vi "Sensor Scaling.vi"(8 "error in":errorcluster) -> (0 "error out":errorcluster, 3 "Output":cluster{"X":dbl[], "Y":dbl[], "Avg point":i16}[](array[cluster]))   [LabVIEW 2015]
uses:
  <vilib>/Analysis/NI_AALPro.lvlib
panel:
  in  "Avg Point":i16=1 min=1 max=500
  out "Offset":dbl format="%0.2f"
  out "Slope":dbl format="%0.2f"
  in  "Unit":string
  in  "Sensor":u16(ring) items=["Load Cell", "LVDT", "LOadcell1", "wq", "load3", "LVDT3", "gggh"]
  in  "Next":bool
  in  "Input Values":dbl[](array[numeric])
  in  "New Calibration":dbl[](array[numeric])
  in  "Sensor Add":bool
  in  "Graph Plot":bool
  in  "Help Button":bool
  in  "Quit":bool
  in  "Save":bool
  out "XY Graph":T1(graph)
  out "error out 2":errorcluster
  out "Numeric":dbl
  out "Old Calibration":dbl[](array[numeric])
  # "Sensor Calibration"
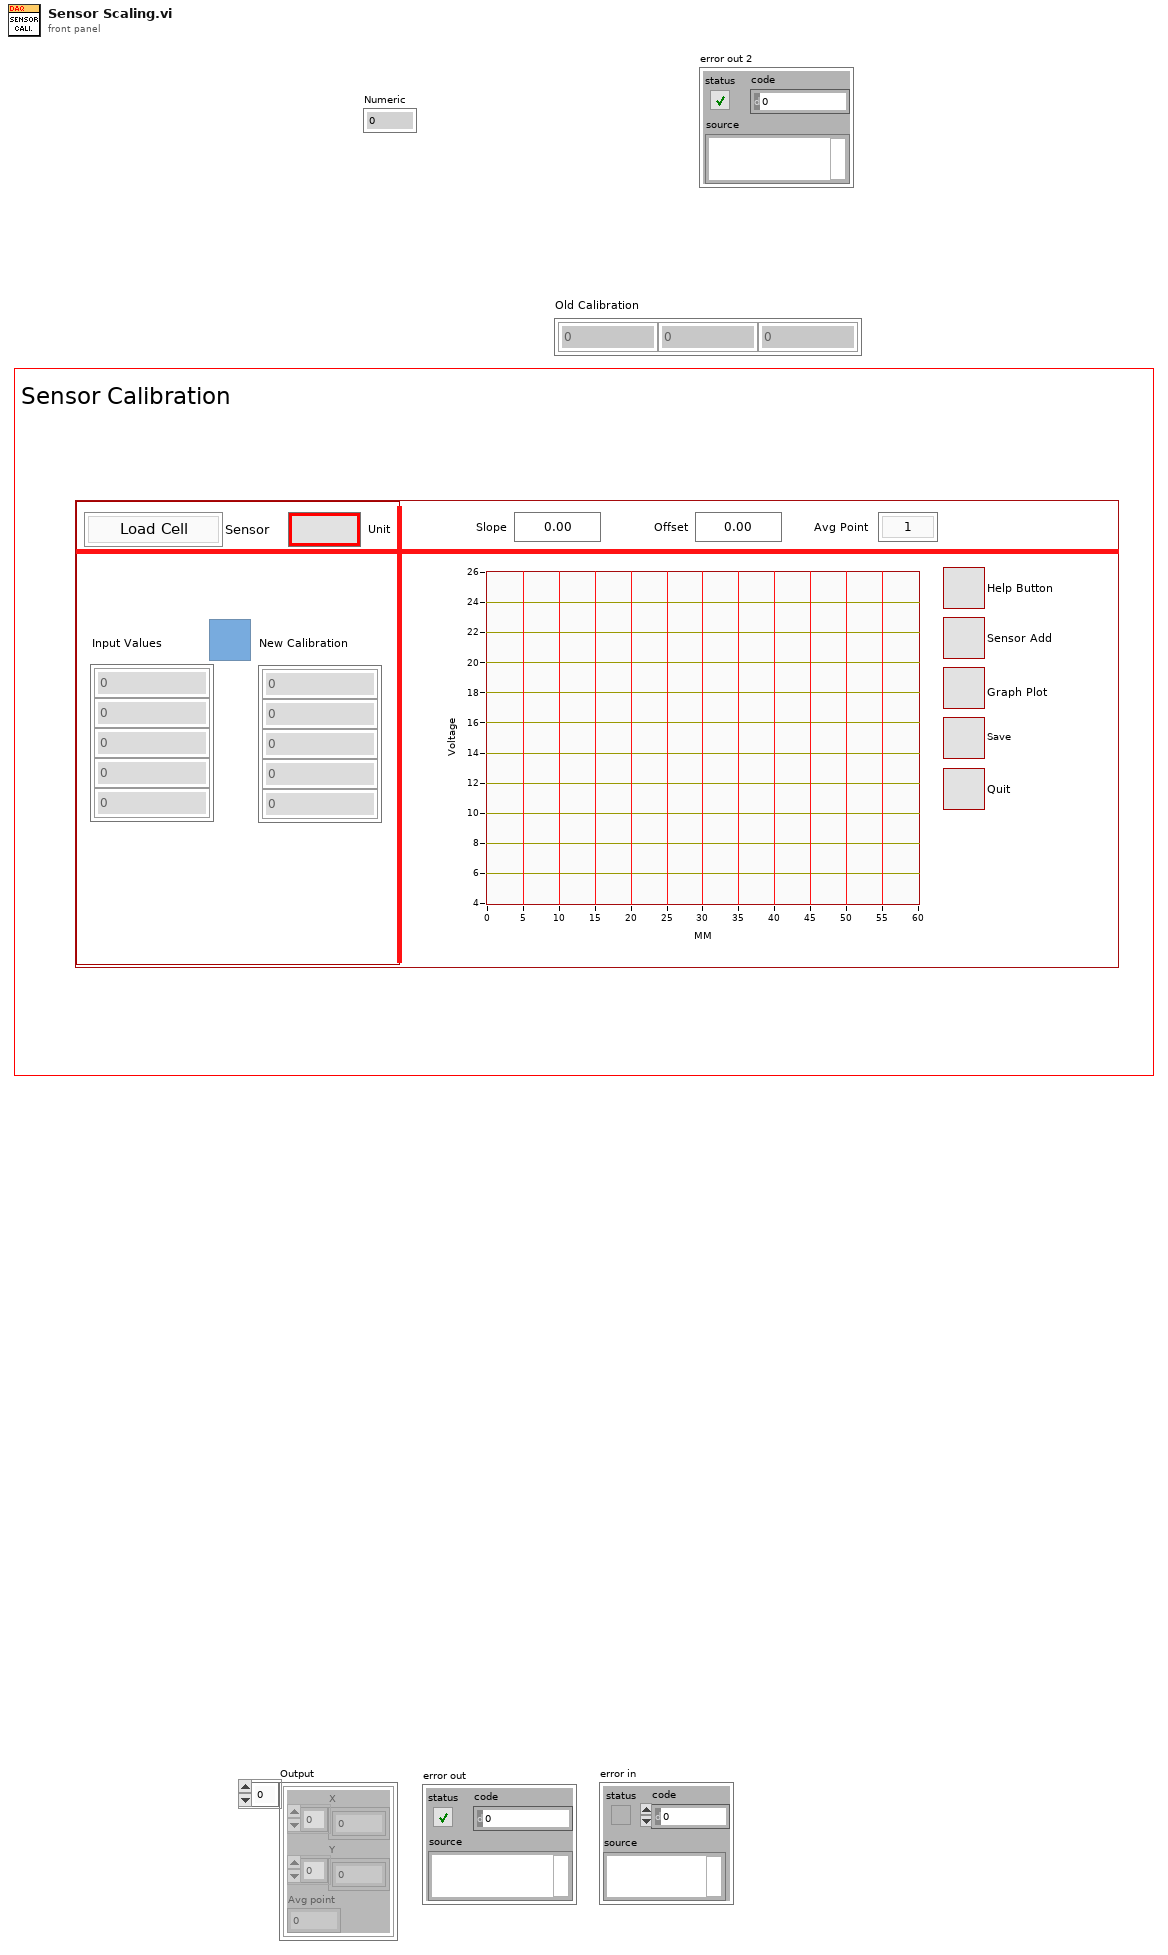
[diagram p1: front panel]
types:
  T1 = cluster{"Input Values":dbl[], "New Calibration":dbl[]}
  T2 = cluster{"XInput":dbl[], "Y New Value":dbl[], "Avg point":i16}[]
  T3 = cluster{"XInput":dbl[], "Y New Value":dbl[], "Avg point":i16}
  T4 = cluster{"Input Values":dbl[], "New Calibration":dbl[], "Sensor":u16}
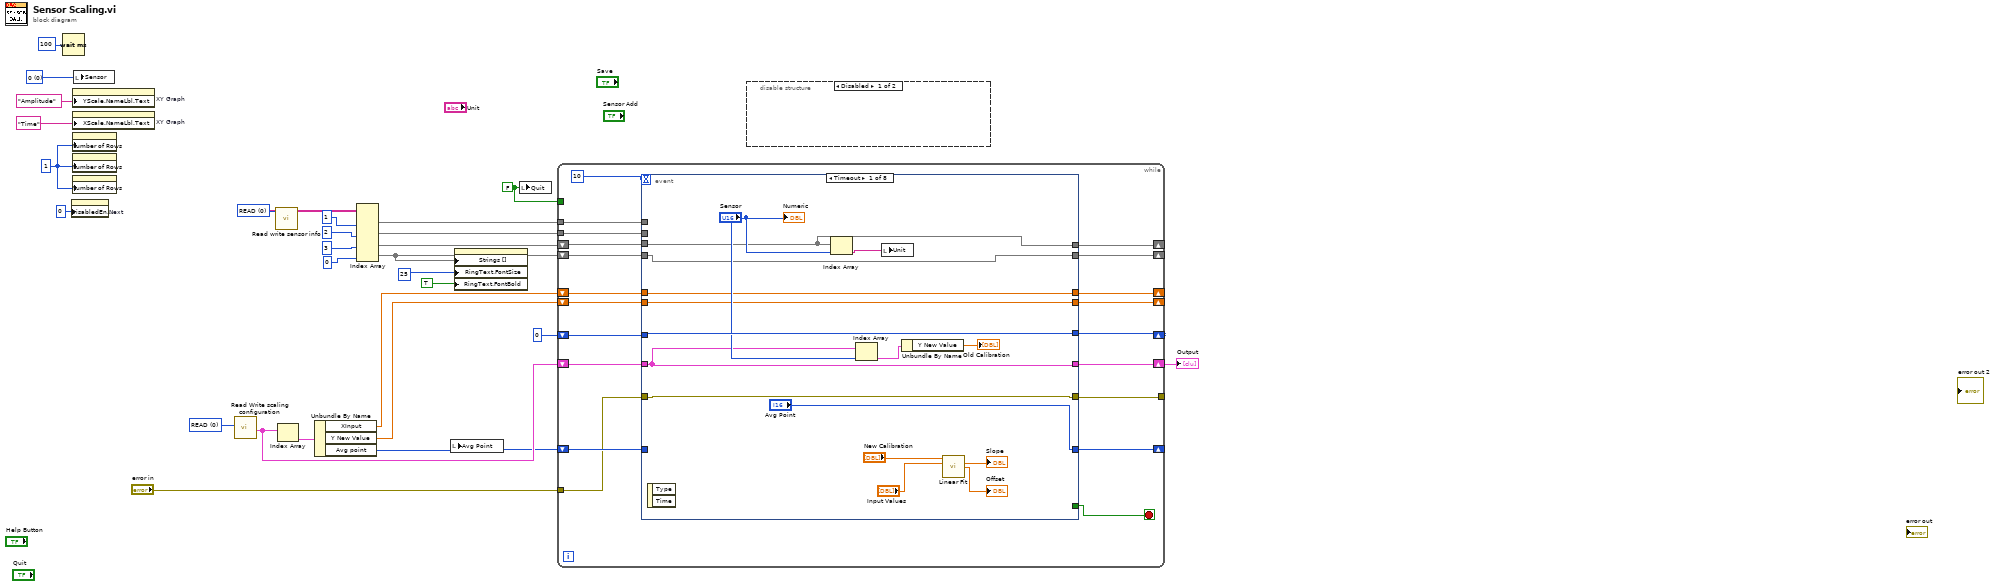
[diagram p0: block diagram]
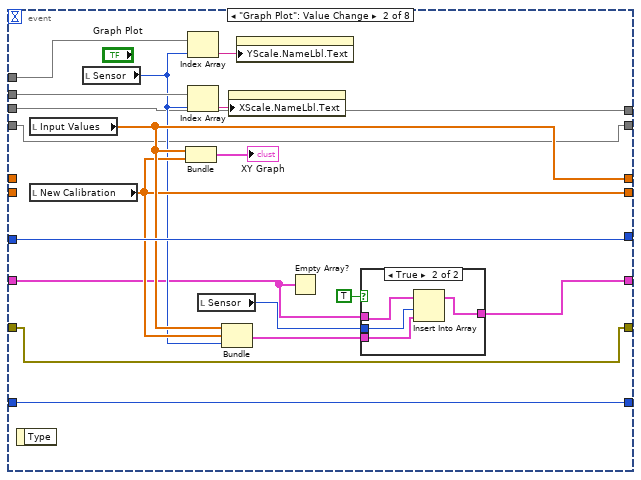
[diagram p3: hidden frame]
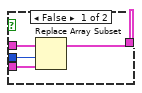
[diagram p4: hidden frame]
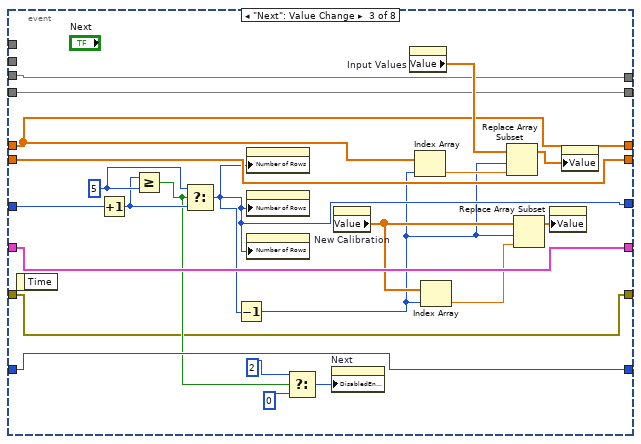
[diagram p5: hidden frame]
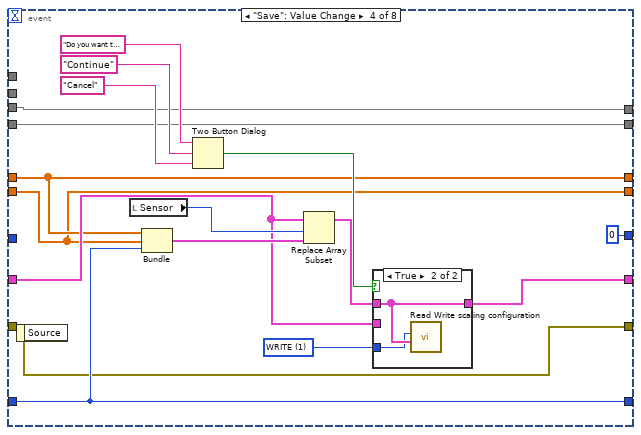
[diagram p6: hidden frame]
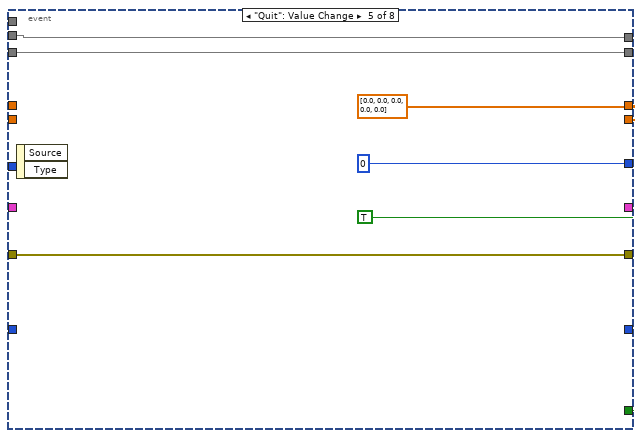
[diagram p8: hidden frame]
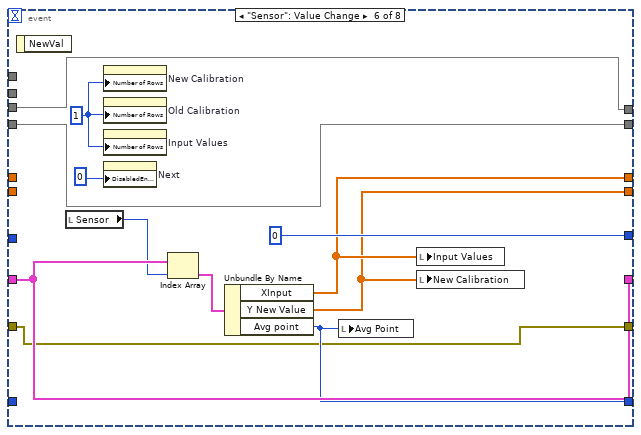
[diagram p9: hidden frame]
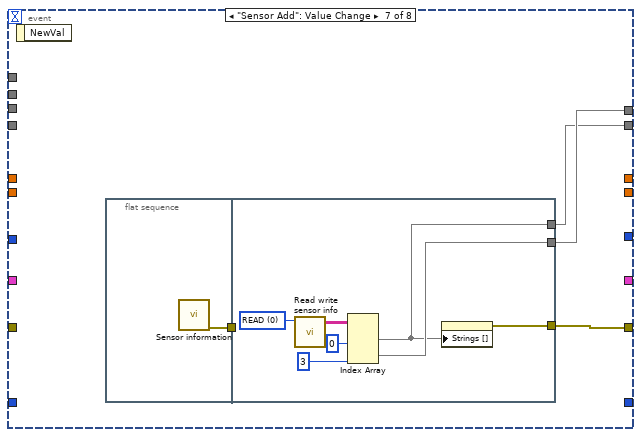
[diagram p10: hidden frame]
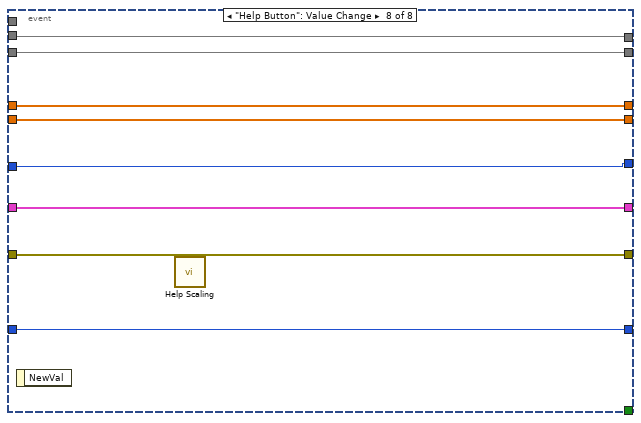
[diagram p11: hidden frame]
diagram:
  w3 = FALSE ("Quit")
  w13 = u16 0 items=["READ", "WRITE"] ("Read/Write")
  w19 = u16 0 items=["READ", "WRITE"] ("Read/Write")
  w9 = u32 1 ("Number of Rows")
  w27 = u16 0 items=["0", "1", "2", "3", "4", "5", "6", "7", "8", "9", "10", "11", "12", "13", "14", "15", "16", "17", "18", "19", "20", "21", "22", "23", "24", "25", "26", "27", "28", "29"] ("Ring")
  n1 = Wait (ms)(milliseconds to wait=u32 100) -> ()  [unwired: 1 out]
  n2 = property on="Next" class="Bool"("DisabledEnum"=u16 0) -> ()  [unwired: 2 in, 2 out]
  n3 = property on="XY Graph" class="XYGraph (strict)"("YScale.NameLbl.Text"="Amplitude" ("Y Scale.Name Label.Text")) -> ()  [unwired: 2 in, 2 out]
  n4 = property on="XY Graph" class="XYGraph (strict)"("XScale.NameLbl.Text"="Time" ("X Scale.Unit Label.Text")) -> ()  [unwired: 2 in, 2 out]
  n5 = property on="Old Calibration" class="Arr (strict)"("Number of Rows"=w9) -> ()  [unwired: 2 in, 2 out]
  n6 = property on="Input Values" class="Arr (strict)"("Number of Rows"=w9) -> ()  [unwired: 2 in, 2 out]
  n7 = property on="New Calibration" class="Arr (strict)"("Number of Rows"=w9) -> ()  [unwired: 2 in, 2 out]
  n8 = local write "Sensor"(w27) -> ()
  n9 = call "Read Write scaling configuration.vi"("Read/Write"=w19) -> ("Output"=w17:T2)  [unwired: 4 in, 2 out]
  n10 = call "Read write sensor info.vi"("Read/Write"=w13) -> ("Table Control out"=w12:string[][])  [unwired: 9 in, 1 out]
  n11 = Index Array(array=w17) -> (element=w18:T3)  [unwired: 1 in]
  n12 = Unbundle By Name(w18) -> ("XInput"=w7:dbl[], "Y New Value"=w6:dbl[], "Avg point"=w16:i16)
  n13 = Index Array(array=w12, index (col) #1=1 ("disabled index (col)"), index (col) #2=2 ("index (row)"), index (col) #3=3 ("index (row)"), index (col) #4=0 ("index (row)")) -> (element #1=w24:string[], element #2=w23:string[], element #3=w5:string[], element #4=w4:string[])  [unwired: 4 in]
  n14 = local write "Avg Point"(w16) -> ()
  n15 = property on="Sensor" class="Ring (strict)"("Strings []"=w4, "RingText.FontSize"=u32 25 ("Ring Text.Font:Size"), "RingText.FontBold"=TRUE ("Ring Text.Font:Bold")) -> ()  [unwired: 2 in, 2 out]
  n16 = local write "Quit"(w3) -> ()
  n17 = while {
    shift-right: [w46] -> _
    shift-left: i8 0 -> [w47]
    shift-right: [w45] -> _
    shift-left: w6 -> [w44]
    tunnel: w24 -> [w42]
    tunnel: w23 -> [w41]
    shift-right: [w40] -> _
    shift-left: w7 -> [w39]
    shift-right: [w37] -> w15
    shift-left: w17 -> [w38]
    shift-right: [w36] -> _
    shift-left: w16 -> [w35]
    tunnel: [w33] -> _
    tunnel: "error in" -> [w30]
    shift-right: [w32] -> _
    shift-left: w5 -> [w31]
    shift-right: [w29] -> _
    shift-left: w4 -> [w34]
    tunnel: w3 -> [_]
    stop <- w43 stop-if-true
    n18 = event shown="[0] Timeout" {
      selector: _ -> [_ _ _ _ _ _ _ _]
      dyn-events: _ -> [_ _ _ _ _ _ _ _]
      timeout: 10 -> [_ _ _ _ _ _ _ _]
      tunnel: [_ _ _ _ TRUE _ _ _] -> w43
      tunnel: w47 -> [w64 w78 w112 _ _ _ _ w165]
      tunnel: [w64 w78 w102 i8 0 i8 0 i8 0 ("y") _ w165] -> w46
      tunnel: [w58 w72 w108 w117 w136 w142 _ w168] -> w45
      tunnel: w44 -> [w58 _ w108 w117 _ _ _ w168]
      tunnel: w42 -> [_ w82 _ _ _ _ _ _]
      tunnel: w41 -> [_ w81 _ _ _ _ _ _]
      tunnel: w31 -> [w53 w67 w93 w115 w135 w141 _ w170]
      tunnel: [w59 w73 w105 w118 w136 w143 _ w169] -> w40
      tunnel: w39 -> [w59 _ w105 w118 _ _ _ w169]
      tunnel: w38 -> [w60 w69 w109 w120 _ w149 _ w167]
      tunnel: [w60 w70 w109 w124 _ w149 _ w167] -> w37
      tunnel: ["Avg Point" w77 w101 w121 _ w146 _ w166] -> w36
      tunnel: w35 -> [_ w77 w101 w121 _ _ _ w166]
      tunnel: w34 -> [w51 w65 w91 w113 w133 w139 _ w163]
      tunnel: [w52 w66 w92 w114 w134 w140 w153 w164] -> w33
      tunnel: [w53 w67 w93 w115 w135 w141 w152 w170] -> w32
      tunnel: w30 -> [w52 w66 w92 w114 w134 w140 _ w164]
      tunnel: [w51 w65 w91 w113 w133 w139 w151 w163] -> w29
      event Timeout {
        n19 = event-data() -> ()  [unwired: 3 out]
        n20 = Index Array(array=w53, index="Sensor") -> (element=w50:string)
        n21 = Index Array(array=w60, index="Sensor") -> (element=w62:T3)
        n22 = local write "Unit"(w50) -> ()
        n23 = Unbundle By Name(w62) -> ("Y New Value"=→"Old Calibration":dbl[])
        n24 = call <vilib>:"Linear Fit.vi"("Y"="New Calibration", "X"="Input Values") -> ("slope"=→"Slope":dbl, "intercept"=→"Offset":dbl)  [unwired: 9 in, 3 out]
        "Numeric" <- "Sensor"
      }
      event "Graph Plot": Value Change {
        n25 = event-data() -> ()  [unwired: 2 out]
        n26 = local read "Input Values"() -> (w73:dbl[])
        n27 = local read "New Calibration"() -> (w72:dbl[])
        n28 = local read "Sensor"() -> (w71:u16)
        n29 = Bundle("Input Values"=w73, "New Calibration"=w72) -> (→"XY Graph":T1)  [unwired: 1 in]
        n30 = Index Array(array=w82, index=w71) -> (element=w80:string)
        n31 = Index Array(array=w81, index=w71) -> (element=w79:string)
        n32 = local read "Sensor"() -> (w74:u16)
        n33 = Bundle("Input Values"=w73, "New Calibration"=w72, "Sensor"=w71) -> (w75:T4)  [unwired: 1 in]
        n34 = property on="XY Graph" class="XYGraph (strict)"("XScale.NameLbl.Text"=w79) -> ()  [unwired: 2 in, 2 out]
        n35 = property on="XY Graph" class="XYGraph (strict)"("YScale.NameLbl.Text"=w80) -> ()  [unwired: 2 in, 2 out]
        n36 = Empty Array?(array=w69) -> ()  [unwired: 1 out]
        n37 = case shown="True" TRUE {
          tunnel: w75 -> [w86 w88]
          tunnel: w74 -> [w85 w90]
          tunnel: w69 -> [w84 w89]
          tunnel: [w83 w87] -> w70
          frame False {
            n38 = Replace Array Subset(array=w84, new element=w86, index=w85) -> (w83:T2)
          }
          frame True {
            n39 = Insert Into Array(array=w89, index=w90, new element=w88) -> (w87:T2)
          }
        }
      }
      event "Next": Value Change {
        w111 = i8 5 ("y")
        n40 = event-data() -> ()  [unwired: 2 out]
        n41 = Increment(x=w112) -> (x+1=w110:i8)
        n42 = Greater Or Equal?(x=w110, y=w111) -> (x >= y?=w100:bool)
        n43 = Select(t=w111, s=w100, f=w110) -> (s? t:f=w102:i8)
        n44 = Decrement(x=w102) -> (x-1=w95:i8)
        n45 = property on="New Calibration" class="Arr (strict)"("Number of Rows"=w102) -> ()  [unwired: 2 in, 2 out]
        n46 = property on="Old Calibration" class="Arr (strict)"("Number of Rows"=w102) -> ()  [unwired: 2 in, 2 out]
        n47 = property on="Input Values" class="Arr (strict)"("Number of Rows"=w102) -> ()  [unwired: 2 in, 2 out]
        n48 = Select(t=2, s=w100, f=0) -> (s? t:f=w97:i32)
        n49 = property on="Next" class="Bool"("DisabledEnum"=w97) -> ()  [unwired: 2 in, 2 out]
        n50 = property on="New Calibration" class="Arr (strict)"() -> ("Value"=w96:dbl[])  [unwired: 2 in, 2 out]
        n51 = property on="Input Values" class="Arr (strict)"() -> ("Value"=w106:dbl[])  [unwired: 2 in, 2 out]
        n52 = Index Array(array=w105, index=w95) -> (element=w104:dbl)
        n53 = Index Array(array=w96, index=w95) -> (element=w94:dbl)
        n54 = Replace Array Subset(array=w106, new element=w104, index=w95) -> (w107:dbl[])
        n55 = Replace Array Subset(array=w96, new element=w94, index=w95) -> (w103:dbl[])
        n56 = property on="New Calibration" class="Arr (strict)"("Value"=w103) -> ()  [unwired: 2 in, 2 out]
        n57 = property on="Input Values" class="Arr (strict)"("Value"=w107) -> ()  [unwired: 2 in, 2 out]
      }
      event "Save": Value Change {
        w116 = u16 1 items=["READ", "WRITE"] ("Read/Write")
        n58 = event-data() -> ()  [unwired: 2 out]
        n59 = local read "Sensor"() -> (w123:u16)
        n60 = Bundle("XInput"=w118, "Y New Value"=w117, "Avg point"=w121) -> (w122:T3)  [unwired: 1 in]
        n61 = Two Button Dialog(message="Do you want to save new calibration value?", 1:"Cancel" ("T button name (\"OK\")"), 2:"Continue" ("F button name (\"Cancel\")")) -> (T button?=w125:bool)
        n62 = Replace Array Subset(array=w120, new element=w122, index=w123) -> (w119:T2)
        n63 = case shown="True" w125 {
          tunnel: w119 -> [_ w132]
          tunnel: [w130 w132] -> w124
          tunnel: w120 -> [w130 _]
          tunnel: w116 -> [_ w131]
          frame False {
          }
          frame True {
            n64 = call "Read Write scaling configuration.vi"("Input"=w132, "Read/Write"=w131) -> ()  [unwired: 3 in, 3 out]
          }
        }
      }
      event "Quit": Value Change {
        w136 = dbl[] [0.0, 0.0, 0.0, 0.0, 0.0]
        n65 = event-data() -> ()  [unwired: 3 out]
      }
      event "Sensor": Value Change {
        w144 = u32 1 ("Number of Rows")
        n66 = event-data() -> ()  [unwired: 2 out]
        n67 = local read "Sensor"() -> (w147:u16)
        n68 = property on="New Calibration" class="Arr (strict)"("Number of Rows"=w144) -> ()  [unwired: 2 in, 2 out]
        n69 = property on="Old Calibration" class="Arr (strict)"("Number of Rows"=w144) -> ()  [unwired: 2 in, 2 out]
        n70 = property on="Input Values" class="Arr (strict)"("Number of Rows"=w144) -> ()  [unwired: 2 in, 2 out]
        n71 = property on="Next" class="Bool"("DisabledEnum"=0) -> ()  [unwired: 2 in, 2 out]
        n72 = Index Array(array=w149, index=w147) -> (element=w150:T3)
        n73 = Unbundle By Name(w150) -> ("XInput"=w143:dbl[], "Y New Value"=w142:dbl[], "Avg point"=w146:i16)
        n74 = local write "Avg Point"(w146) -> ()
        n75 = local write "Input Values"(w143) -> ()
        n76 = local write "New Calibration"(w142) -> ()
      }
      event "Sensor Add": Value Change {
        n77 = event-data() -> ()  [unwired: 2 out]
        n78 = flat-sequence {
          tunnel: [w155] -> w154
          tunnel: w154 -> [_]
          tunnel: [w159] -> w153
          tunnel: [w157] -> w152
          tunnel: [w156] -> w151
          frame #0 {
            n79 = call "Sensor information.vi"() -> ("error in (no error) 2"=w155:errorcluster)  [unwired: 11 in]
          }
          frame #1 {
            w162 = u16 0 items=["READ", "WRITE"] ("Read/Write")
            n80 = call "Read write sensor info.vi"("Read/Write"=w162) -> ("Table Control out"=w161:string[][])  [unwired: 9 in, 1 out]
            n81 = Index Array(array=w161, index (col) #1=0 ("disabled index (col)"), index (col) #2=3 ("index (col)")) -> (element #1=w156:string[], element #2=w157:string[])  [unwired: 2 in]
            n82 = property on="Sensor" class="Ring (strict)"("Strings []"=w156) -> (error out=w159:errorcluster)  [unwired: 2 in, 1 out]
          }
        }
      }
      event "Help Button": Value Change {
        n83 = event-data() -> ()  [unwired: 2 out]
        n84 = call "Help Scaling.vi"() -> ()  [unwired: 12 in]
      }
    }
  }
  "Output" <- w15
  n85 = disable-structure shown="Disabled" {
    frame Disabled {
    }
    frame Enabled {
    }
  }
